vi "borrar.vi"() -> ()   [LabVIEW 2018]
panel:
  in  "Clave":string
  in  "Array":string[](array[string])
  in  "usuario":string
  out "spreadsheet string":string
  out "array w/ subset deleted":string[][](array[string])
  out "before substring 3":string
  out "match substring 3":string
  out "after substring 3":string
  out "array 2":string[][](array[string])
  out "element 3":string
  out "text 2":string
  in  "OK Button":bool
  in  "stop":bool
  out "appended path":path
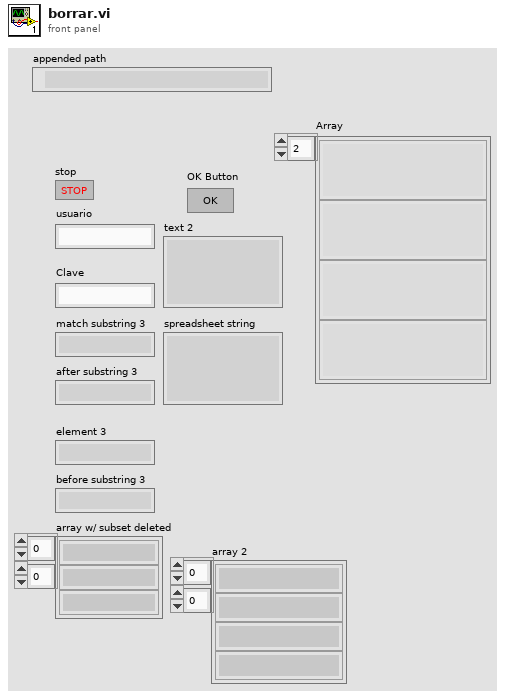
[diagram p1: front panel]
types:
  T1 = enum16{"open", "replace", "create", "open or create", "replace or create", "replace or create with confirmation"}
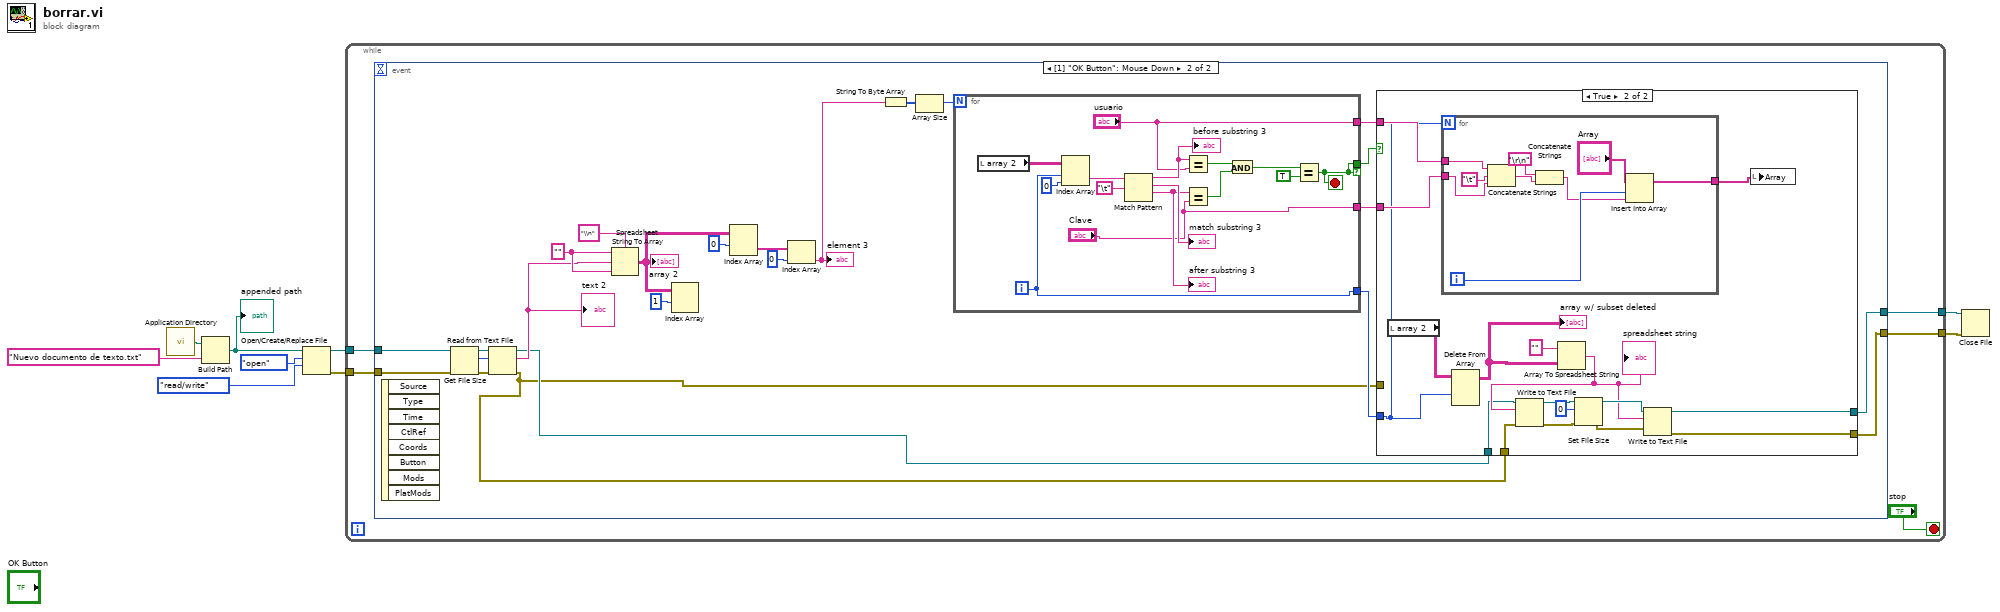
[diagram p0: block diagram]
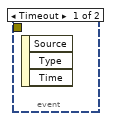
[diagram p2: hidden frame]
diagram:
  n1 = call <vilib>:"Application Directory.vi"() -> ("Application Directory"=w9:path)
  n2 = Build Path(base path=w9, name or relative path="Nuevo documento de texto.txt") -> (appended path=w8:path)
  "appended path" <- w8
  n3 = Open/Create/Replace File(file path (use dialog)=w8, operation (0:open)=T1."open", access (0:read/write)=enum16{"read/write", "read-only", "write-only"}."read/write") -> (refnum out=w4:refnum<file>, error out=w5:errorcluster)  [unwired: 3 in, 1 out]
  n4 = while {
    tunnel: w5 -> [w13]
    tunnel: w4 -> [w12]
    tunnel: [w11] -> w2
    tunnel: [w10] -> w1
    stop <- "stop" stop-if-true
    n5 = event shown="[1] \"OK Button\": Mouse Down" {
      selector: _ -> [_ _]
      dyn-events: _ -> [_ _]
      timeout: _ -> [_ _]
      tunnel: w13 -> [_ w23]
      tunnel: w12 -> [_ w35]
      tunnel: [_ w19] -> w11
      tunnel: [_ w18] -> w10
      event Timeout {
        n6 = event-data() -> ()  [unwired: 1 in, 3 out]
      }
      event "OK Button": Mouse Down {
        w27 = "" ("format string")
        n7 = event-data() -> ()  [unwired: 1 in, 8 out]
        n8 = Get File Size(file=w35, error in=w23) -> (refnum out=w37:refnum<file>, size (in bytes)=w38:i64, 0:w36:errorcluster)
        n9 = Read from Text File(file (use dialog)=w37, count=w38, error in=w36) -> (refnum out=w22:refnum<file>, text=w26:string, error out=w15:errorcluster)  [unwired: 1 in, 1 out]
        "text 2" <- w26
        n10 = Spreadsheet String To Array(delimiter (Tab)="\\n", format string=w27, spreadsheet string=w26, array type (2D Dbl)=w27) -> (array=w32:string[][])
        "array 2" <- w32
        n11 = Index Array(array=w32, index (row)=1) -> ()  [unwired: 1 in, 1 out]
        n12 = Index Array(array=w32, index (row)=0) -> (element=w33:string[])  [unwired: 1 in]
        n13 = Index Array(array=w33, index=0) -> (element=w25:string)
        "element 3" <- w25
        n14 = String To Byte Array(string=w25) -> (unsigned byte array=w34:u8[])
        n15 = Array Size(array=w34) -> (size(s)=w24:i32)
        n16 = for {
          N: w24 -> [_]
          tunnel: [w42] -> w20 if=w42
          tunnel: [w43] -> w21
          tunnel: ["Clave"] -> w17
          tunnel: ["usuario"] -> w16
          i -> [w43]
          stop <- w42 stop-if-true
          n17 = local read "array 2"() -> (w41:string[][])
          n18 = Index Array(array=w41, index (row)=w43, index (col)=0 ("disabled index (col)")) -> (element=w52:string)
          n19 = Match Pattern(string=w52, regular expression="\t") -> (before substring=w48:string, match substring=→"match substring 3":string, after substring=w49:string)  [unwired: 1 in, 1 out]
          "before substring 3" <- w48
          "after substring 3" <- w49
          n20 = Equal?(x=w48, y="usuario") -> (x = y?=w47:bool)
          n21 = Equal?(x=w49, y="Clave") -> (x = y?=w46:bool)
          n22 = And(x=w47, y=w46) -> (x .and. y?=w45:bool)
          n23 = Equal?(x=w45, y=TRUE) -> (x = y?=w42:bool)
        }
        n24 = case shown="True" w20 {
          tunnel: w21 -> [_ w55]
          tunnel: [_ w67] -> w19
          tunnel: [_ w66] -> w18
          tunnel: w22 -> [_ w60]
          tunnel: w15 -> [_ w59]
          tunnel: w17 -> [_ w56]
          tunnel: w16 -> [_ w57]
          tunnel: w15 -> [_ _]
          frame False {
          }
          frame True {
            n25 = local read "array 2"() -> (w70:string[][])
            n26 = for {
              N: w55 -> [_]
              tunnel: w57 -> [w79]
              tunnel: w56 -> [w77]
              tunnel: [w74] -> w54
              i -> [w73]
              n27 = Concatenate Strings(w79, "\t", w77) -> (w75:string)
              n28 = Concatenate Strings("\r\n", w75) -> (w72:string)
              n29 = Insert Into Array "Insert Into Array"(array="Array", index=w73, new element=w72) -> (w74:string[])
            }
            n30 = Delete From Array "Delete From Array"(array=w70, index (row)=w55) -> (array with subset deleted=w69:string[][])  [unwired: 2 in, 1 out]
            "array w/ subset deleted" <- w69
            n31 = Array To Spreadsheet String(array=w69, 3:"" ("format string")) -> (spreadsheet string=w61:string)  [unwired: 1 in]
            "spreadsheet string" <- w61
            n32 = Write to Text File(file (use dialog)=w60, text=w61, error in=w59) -> (refnum out=w63:refnum<file>, error out=w62:errorcluster)  [unwired: 1 in, 1 out]
            n33 = Set File Size(4:w62, 6:i64 0 ("size (in bytes)"), 7:w63) -> (0:w64:errorcluster, 3:w65:refnum<file>)
            n34 = Write to Text File(file (use dialog)=w65, text=w61, error in=w64) -> (refnum out=w67:refnum<file>, error out=w66:errorcluster)  [unwired: 1 in, 1 out]
            n35 = local write "Array"(w54) -> ()
          }
        }
      }
    }
  }
  n36 = Close File(refnum=w2, error in=w1) -> ()  [unwired: 2 out]
